vi "CANOpen_Main.vi"() -> ()   [LabVIEW 2021, in "CANOpen Addon Engine.lvlib"]
uses:
  CANOpen Addon Engine.lvlib
  SubVIS/CANOpen_Settings.ctl
  SubVIS/CANOpen_Node Settings.ctl
  Shared/CANOpen_Bus Settings.ctl
  Shared/CANOpen Interface Name.ctl
  <vilib>/CANopenLib/CANOPEN.llb/CANopen BaudRate.ctl
  SubVIS/CANOpen_Node Message Settings.ctl
  Shared/CANOpen_PDO Settings.ctl
  Shared/CANOpen_PDO Parameter Settings.ctl
  Shared/CANOpen_PDO Data Type.ctl
  Shared/CANopen Byte Order.ctl
  Shared/CANOpen_SDO Settings.ctl
  SubVIS/CANOpen_NMT Settings.ctl
  Shared/CanOpen_NMT_Config.ctl
  Shared/CanOpen_NMT_Static detect.ctl
  SubVIs/CanOpen_Main Node Ids.ctl
  SubVIS/CANOpen_VS Data Refs.ctl
  <vilib>/NI VeriStand/Custom Device API/Data Reference.ctl
  <vilib>/NI VeriStand/Custom Device API/Block Data Reference.ctl
  SubVIS/CANOpen_VS Bidirectional Data Refs.ctl
  SubVIS/CANOpen_VS SDOs Data Refs.ctl
  SubVIs/CanOpen_SDO Dynamic queue.ctl
  Shared/CANOpen_SDO queue W data.ctl
  Shared/CANOpen_SDO queue mode.ctl
  Shared/CANOpen_PDO Data Type in queue.ctl
  SubVIS/CANOpen_VS Status Management Data Refs.ctl
  SubVIs/CanOpen_NMT_HWOut_ChannelPairs.ctl
  SubVIs/CanOpen_NMT_HWIn_ChannelPairs.ctl
  <vilib>/NI VeriStand/Custom Device API/Custom Device Timed Loop Priority.ctl
  <vilib>/Platform/TimedLoop/XDataNode/timing_clust.ctl
  <vilib>/Platform/TimedLoop/XDataNode/nitl_modes.ctl
  <vilib>/Platform/TimedLoop/XDataNode/wakeup.ctl
  SubVIs/CanOpen_Main States.ctl
  SubVIs/CANOpen_Main_Close xPDOs.vi
  SubVIs/CANOpen_Main_Close HB NG EM.vi
  SubVIs/CANOpen_State_Opp_Preopp.vi
  SubVIs/CANOpen_Main_Compare RPDO Data for Change.vi
  <vilib>/CANopenLib/CANOPEN.llb/CANopen Interface Create.vi
  SubVIs/CANOpen_Check_Node_State for Node without HB NG.vi
  <vilib>/CANopenLib/CANOPEN.llb/CANopen Error Control Read.vi
  <vilib>/CANopenLib/CANOPEN.llb/CANopen Heartbeat State Read.vi
  <vilib>/CANopenLib/CANOPEN.llb/CANopen Node Guarding State Read.vi
  <vilib>/CANopenLib/CANOPEN.llb/CANopen Emergency Read.vi
  SubVIs/CANOpen_Main_Prepare status data.vi
  SubVIs/CANOpen_Main_Scale RPDO Data.vi
  <vilib>/CANopenLib/CANOPEN.llb/CANopen RPDO Write.vi
  <vilib>/CANopenLib/CANOPEN.llb/CANopen TPDO Read.vi
  SubVIs/CANOpen_Main_Scale TPDO Data.vi
  <vilib>/CANopenLib/CANOPEN.llb/CANopen Close.vi
  <vilib>/CANopenLib/CANOPEN.llb/CANopen SYNC Close.vi
  <vilib>/CANopenLib/CANOPEN.llb/CANopen RPDO Close.vi
  <vilib>/CANopenLib/CANOPEN.llb/CANopen TPDO Close.vi
  <vilib>/CANopenLib/CANOPEN.llb/CANopen SDO Create.vi
  <vilib>/CANopenLib/CANOPEN.llb/CANopen SDO Write.vi
  <vilib>/CANopenLib/CANOPEN.llb/CANopen SDO Write [U16].vi
  <vilib>/CANopenLib/CANOPEN.llb/CANopen SDO Close.vi
  <vilib>/CANopenLib/CANOPEN.llb/CANopen Heartbeat Close.vi
  <vilib>/CANopenLib/CANOPEN.llb/CANopen SDO Write [U8].vi
  <vilib>/CANopenLib/CANOPEN.llb/CANopen Node Guarding Close.vi
  <vilib>/CANopenLib/CANOPEN.llb/CANopen Emergency Close.vi
  SubVIs/CANOpen_Main_Set All Node States.vi
  <vilib>/CANopenLib/CANOPEN.llb/CANopen Interface Close.vi
  <vilib>/Platform/TimedLoop/XDataNode/XDataNode.xnode
  <vilib>/Platform/TimedLoop/XDataNode/XDNodeRunTimeDep.lvlib
  <vilib>/NI VeriStand/Custom Device API/Custom Device API.lvlib
  Shared/CANOpen Addon Shared.lvlib
panel:
  out "Interface Name":T1 caption="CANOpen Interface Name" items=["CANopen01", "CANopen02", "CANopen03", "CANopen04", "CANopen05", "CANopen06", "CANopen07", "CANopen08", "CANopen09", "CANopen10", "CANopen11", "CANopen12", "CANopen13", "CANopen14", "CANopen15", "CANopen16", "CANopen17", "CANopen18", "CANopen19", "CANopen20", "CANopen21", "CANopen22", "CANopen23", "CANopen24", "CANopen25", "CANopen26", "CANopen27", "CANopen28", "CANopen29", "CANopen30", "CANopen31", "CANopen32"]
  in  "Parent":string
  in  "Parameters":T2={"Driver Settings"={"CANOpen Bus Settings"={"CANOpen Interface Name"=0, "Baud Rate"=0, "Termination"=FALSE, "Sync Period (ms)"=10, "Enable 9881"=FALSE, "RIO Device"=0, "Enable SYNC"=FALSE, "Scan & Print"=FALSE}, "Nodes"=[], "Node Ids"=[]}, "Data References"={"Hardware Input"={"FIFO"=refnum, "Channel Pairs"={"Chan Refs"=[], "Prev. Values"=[]}}, "Hardware Output"={"FIFO"=refnum, "Channel Pairs"={"Block Refs"=[], "Prev. Values"=[]}}}, "Bus Commands"={"Hardware Output"={"FIFO"=refnum, "Channel Pairs"={"Chan Refs"=[], "Prev. Values"=[]}}, "Hardware Input"={"FIFO"=refnum}}, "SDO Asynch"={"List SDO"={"FIFO Req"=refnum, "Req Chan."={"Chan Refs"=[], "NodeIndex"=[]}, "FIFO Resp"=refnum, "Resp Chan."={"Chan Refs"=[]}, "Node IDs"=[], "FIFO array"=[]}, "HW Dyn Write"={"FIFO Req"=refnum, "FIFO Resp"=refnum, "Req Chan."={"Chan Refs"=[], "Node IDs"=[]}, "Resp Chan."={"Chan Refs"=[]}}, "HW Dyn Read"={"FIFO Req"=refnum, "FIFO Resp"=refnum, "Req Chan."={"Chan Refs"=[], "Node IDs"=[]}, "Resp Chan."={"Chan Refs"=[]}}}, "Status NMT"={"Hardware Output"={"FIFO"=refnum, "Channel Pairs"={"Chan Refs"=[], "Prev. Values"=[], "Node index"=[]}}, "Hardware Input"={"FIFO"=refnum, "Channel Pairs"={"Chan Refs"=[], "Prev. Values"=[], "Node index"=[]}}}} {"Status NMT"."Hardware Output"."Channel Pairs"."Chan Refs"."Data Reference" format="%.0x"; "Status NMT"."Hardware Input"."Channel Pairs"."Chan Refs" format="%.0x"; "SDO Asynch"."HW Dyn Read"."Resp Chan."."Chan Refs" format="%.0x"; "SDO Asynch"."HW Dyn Read"."Req Chan."."Chan Refs" format="%.0x"; "SDO Asynch"."HW Dyn Write"."Resp Chan."."Chan Refs" format="%.0x"; "SDO Asynch"."HW Dyn Write"."Req Chan."."Chan Refs" format="%.0x"; "SDO Asynch"."List SDO"."Resp Chan."."Chan Refs" format="%.0x"; "SDO Asynch"."List SDO"."Req Chan."."Chan Refs" format="%.0x"; "Bus Commands"."Hardware Output"."Channel Pairs"."Chan Refs" format="%.0x"; "Data References"."Hardware Input"."Channel Pairs"."Chan Refs" format="%.0x"; "Data References"."Hardware Output"."Channel Pairs"."Block Refs"."Data Reference" format="%.0x"; "Driver Settings"."CANOpen Bus Settings"."Baud Rate" items=["1 Mbit/s"=0, "800 kbit/s"=1, "500 kbit/s"=2, "250 kbit/s"=3, "125 kbit/s"=4, "50 kbit/s"=6, "20 kbit/s"=7, "10 kbit/s"=8]; "Driver Settings"."CANOpen Bus Settings"."CANOpen Interface Name" items=["CANopen01", "CANopen02", "CANopen03", "CANopen04", "CANopen05", "CANopen06", "CANopen07", "CANopen08", "CANopen09", "CANopen10", "CANopen11", "CANopen12", "CANopen13", "CANopen14", "CANopen15", "CANopen16", "CANopen17", "CANopen18", "CANopen19", "CANopen20", "CANopen21", "CANopen22", "CANopen23", "CANopen24", "CANopen25", "CANopen26", "CANopen27", "CANopen28", "CANopen29", "CANopen30", "CANopen31", "CANopen32"]; "Driver Settings"."Nodes"."NMT"."Node init static SDO state" items=["start remote node"=1, "enter pre-operational"=128]; "Driver Settings"."Nodes"."NMT"."Node run state" items=["start remote node"=1, "stop remote node"=2, "enter pre-operational"=128, "reset node"=129, "reset communication"=130]; "Driver Settings"."Nodes"."Dynamic SDOs"."Sub-Index (0)" format="%.0x"; "Driver Settings"."Nodes"."Dynamic SDOs"."Object Index" format="%.0x"; "Driver Settings"."Nodes"."Dynamic SDOs"."Block Data" format="%.0x"; "Driver Settings"."Nodes"."RPDOs"."PDO Channel" items=["PDO 1", "PDO 2", "PDO 3", "PDO 4"]; "Driver Settings"."Nodes"."TPDOs"."PDO Channel" items=["PDO 1", "PDO 2", "PDO 3", "PDO 4"]; "Driver Settings"."Nodes"."SDOs"."Sub-Index (0)" format="%.0x"; "Driver Settings"."Nodes"."SDOs"."Object Index" format="%.0x"; "Driver Settings"."Nodes"."SDOs"."Block Data" format="%.0x"}
  in  "stop":bool
  in  "error in":errorcluster
  out "error out":errorcluster
  # "LSB"
  # "MSB"
  # "LSB"
  # "MSB"
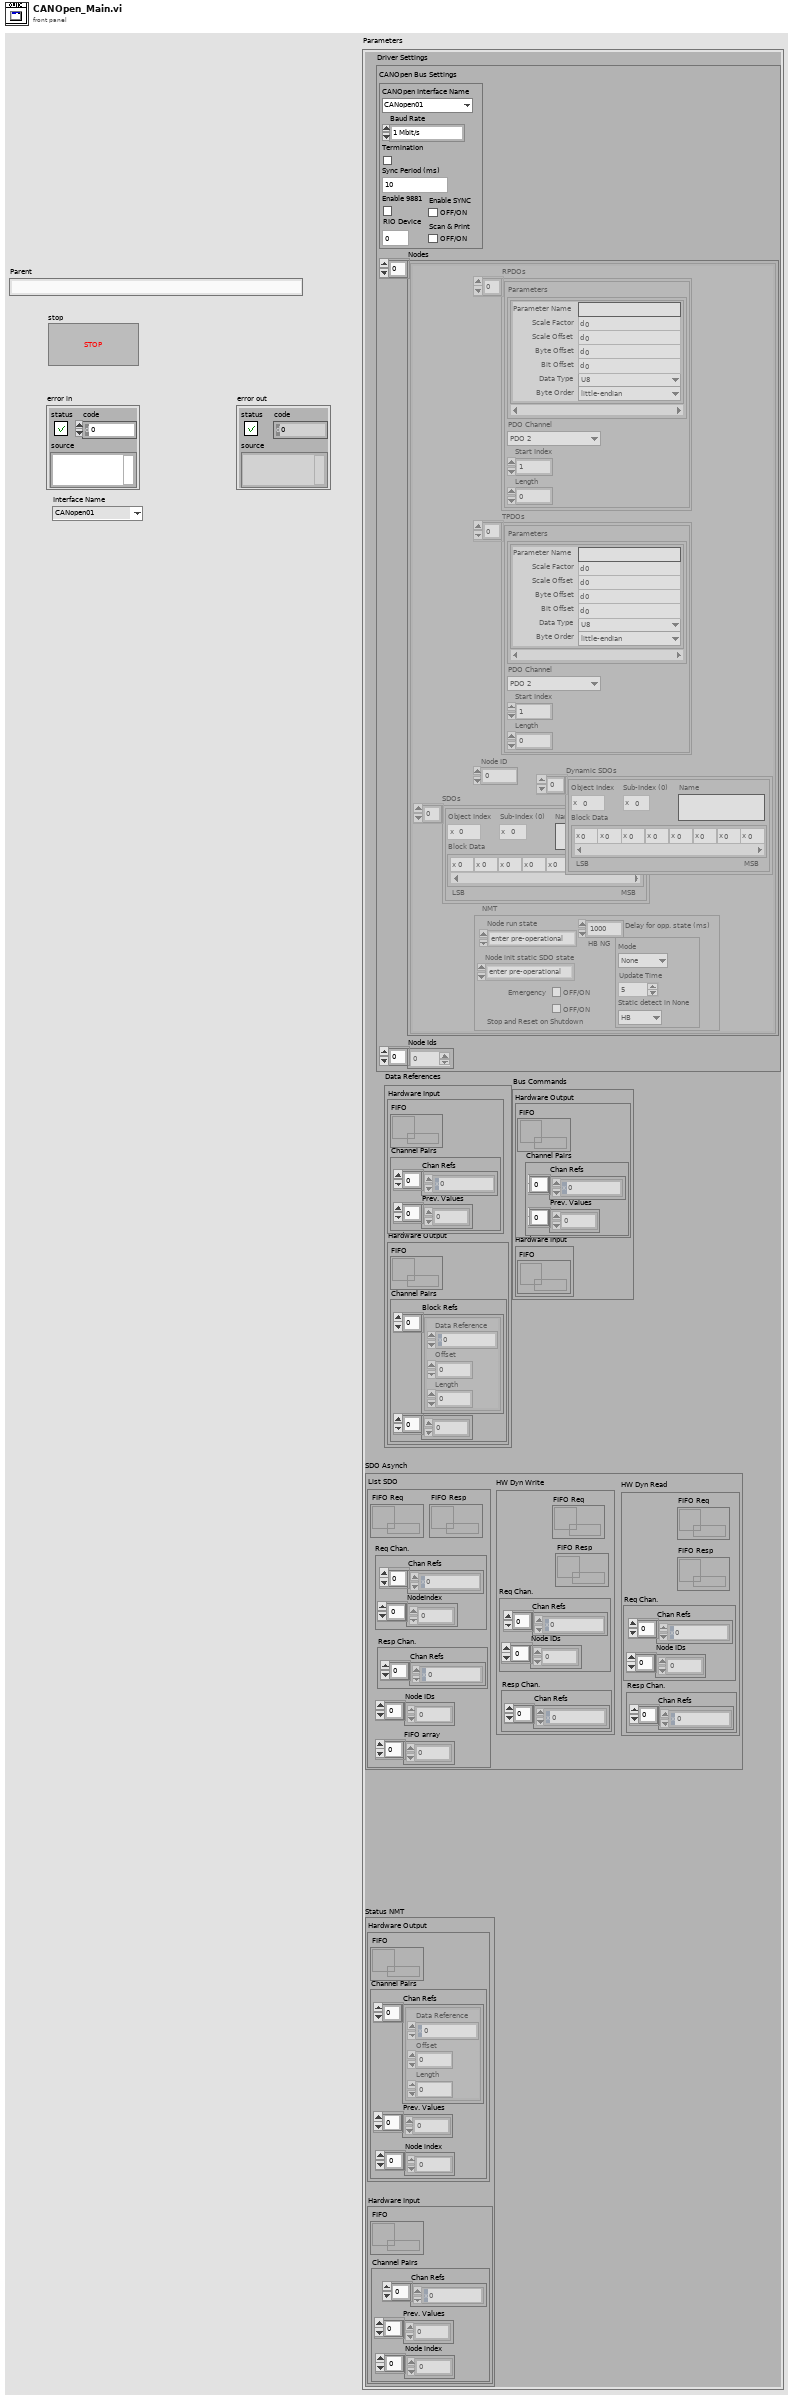
[diagram p1: front panel]
types:
  T1 = typedef "CANOpen Addon Shared.lvlib/CANOpen Interface Name.ctl" = u32
  T2 = typedef "CANOpen Addon Engine.lvlib/CANOpen_Settings.ctl" = cluster{"Driver Settings":T3, "Data References":T16, "Bus Commands":T19, "SDO Asynch":T20, "Status NMT":T21}
  T3 = typedef "CANOpen Addon Engine.lvlib/CANOpen_Node Settings.ctl" = cluster{"CANOpen Bus Settings":T4, "Nodes":T6[], "Node Ids":T15}
  T4 = typedef "CANOpen Addon Shared.lvlib/CANOpen_Bus Settings.ctl" = cluster{"CANOpen Interface Name":T1, "Baud Rate":T5, "Termination":bool, "Sync Period (ms)":i64, "Enable 9881":bool, "RIO Device":u16, "Enable SYNC":bool, "Scan & Print":bool}
  T5 = typedef "CANopen BaudRate.ctl" = u32
  T6 = typedef "CANOpen Addon Engine.lvlib/CANOpen_Node Message Settings.ctl" = cluster{"RPDOs":T7[], "TPDOs":T7[], "Node ID":u8, "SDOs":T11[], "Dynamic SDOs":T11[], "NMT":T12}
  T7 = typedef "CANOpen Addon Shared.lvlib/CANOpen_PDO Settings.ctl" = cluster{"Parameters":T8[], "PDO Channel":u8, "Start Index":u32, "Length":u32}
  T8 = typedef "CANOpen Addon Shared.lvlib/CANOpen_PDO Parameter Settings.ctl" = cluster{"Parameter Name":string, "Scale Factor":dbl, "Scale Offset":dbl, "Byte Offset":u8, "Bit Offset":u8, "Data Type":T9, "Byte Order":T10}
  T9 = typedef "CANOpen Addon Shared.lvlib/CANOpen_PDO Data Type.ctl" = enum16{"U8", "U16", "U32", "I8", "I16", "I32", "Single", "Double", "Boolean"}
  T10 = typedef "CANOpen Addon Shared.lvlib/CANopen Byte Order.ctl" = enum16{"big-endian network order", "little-endian"}
  T11 = typedef "CANOpen Addon Shared.lvlib/CANOpen_SDO Settings.ctl" = cluster{"Object Index":u16, "Sub-Index (0)":u8, "Block Data":u8[], "Name":string}
  T12 = typedef "CANOpen Addon Engine.lvlib/CANOpen_NMT Settings.ctl" = cluster{"Node run state":u16, "Emergency":bool, "HB NG":T13, "Delay for opp. state (ms)":dbl, "Node init static SDO state":u16, "Stop and Reset on Shutdown":bool}
  T13 = typedef "CANOpen Addon Shared.lvlib/CanOpen_NMT_Config.ctl" = cluster{"Mode":T14, "Update Time":u16, "Static detect in None":T14}
  T14 = typedef "CANOpen Addon Shared.lvlib/CanOpen_NMT_Static detect.ctl" = enum16{"None", "HB", "NG"}
  T15 = typedef "CANOpen Addon Engine.lvlib/CanOpen_Main Node Ids.ctl" = u8[]
  T16 = typedef "CANOpen Addon Engine.lvlib/CANOpen_VS Data Refs.ctl" = cluster{"Hardware Input":cluster{"FIFO":refnum<k33>, "Channel Pairs":cluster{"Chan Refs":T17[], "Prev. Values":dbl[]}}, "Hardware Output":cluster{"FIFO":refnum<k33>, "Channel Pairs":cluster{"Block Refs":T18[], "Prev. Values":dbl[]}}}
  T17 = typedef "Custom Device API.lvlib/Data Reference.ctl" = i32
  T18 = typedef "Custom Device API.lvlib/Block Data Reference.ctl" = cluster{"Data Reference":T17, "Offset":u64, "Length":u64}
  T19 = typedef "CANOpen Addon Engine.lvlib/CANOpen_VS Bidirectional Data Refs.ctl" = cluster{"Hardware Output":cluster{"FIFO":refnum<k33>, "Channel Pairs":cluster{"Chan Refs":T17[], "Prev. Values":dbl[]}}, "Hardware Input":cluster{"FIFO":refnum<k33>}}
  T20 = typedef "CANOpen Addon Engine.lvlib/CANOpen_VS SDOs Data Refs.ctl" = cluster{"List SDO":cluster{"FIFO Req":refnum<k33>, "Req Chan.":cluster{"Chan Refs":T17[], "NodeIndex":dbl[]}, "FIFO Resp":refnum<k33>, "Resp Chan.":cluster{"Chan Refs":T17[]}, "Node IDs":u8[], "FIFO array":dbl[]}, "HW Dyn Write":cluster{"FIFO Req":refnum<k33>, "FIFO Resp":refnum<k33>, "Req Chan.":cluster{"Chan Refs":T17[], "Node IDs":u8[]}, "Resp Chan.":cluster{"Chan Refs":T17[]}}, "HW Dyn Read":cluster{"FIFO Req":refnum<k33>, "FIFO Resp":refnum<k33>, "Req Chan.":cluster{"Chan Refs":T17[], "Node IDs":u8[]}, "Resp Chan.":cluster{"Chan Refs":T17[]}}}
  T21 = typedef "CANOpen Addon Engine.lvlib/CANOpen_VS Status Management Data Refs.ctl" = cluster{"Hardware Output":cluster{"FIFO":refnum<k33>, "Channel Pairs":T22}, "Hardware Input":cluster{"FIFO":refnum<k33>, "Channel Pairs":T23}}
  T22 = typedef "CANOpen Addon Engine.lvlib/CanOpen_NMT_HWOut_ChannelPairs.ctl" = cluster{"Chan Refs":T18[], "Prev. Values":dbl[], "Node index":dbl[]}
  T23 = typedef "CANOpen Addon Engine.lvlib/CanOpen_NMT_HWIn_ChannelPairs.ctl" = cluster{"Chan Refs":T17[], "Prev. Values":dbl[], "Node index":dbl[]}
  T24 = typedef "Custom Device API.lvlib/Custom Device Timed Loop Priority.ctl" = enum32{"Low", "Medium", "High"}
  T25 = typedef "CANOpen Addon Engine.lvlib/CanOpen_SDO queue ref.ctl" = cluster{"SDOReq":refnum<queue>}
  T26 = typedef "CANOpen Addon Engine.lvlib/CanOpen_Main States.ctl" = enum16{"NMT", "Device Status", "RPDO", "DYN SDO", "SYNC", "TPDO", "Status"}
  T27 = typedef "XDNodeRunTimeDep.lvlib/timing_clust.ctl" = cluster{"Expected End [f-1]":u64, "Actual End [f-1]":u64, "Finished Late? [f-1]":bool, "Expected End [i-1]":u64, "Actual End [i-1]":u64, "Finished Late? [i-1]":bool, "Expected Start [i]":u64, "Actual Start [i]":u64, "Expected Start [f]":u64, "Actual Start [f]":u64, "Source Name":string, "Structure Name":string, "Period":i64, "Deadline":i64, "Offset":i64, "Start":i64, "Priority":i32, "Timeout":i32, "Mode":T28, "Wakeup Reason":T29, "Error":errorcluster, "Source Type":string, "Secondary Source Type":string, "Global End Time":u64, "Global Start Time":u64, "Frame Duration":u64, "Iteration Duration":u64, "Assigned CPU":i32, "I/O Scan Engine Mode":u32}
  T28 = typedef "XDNodeRunTimeDep.lvlib/nitl_modes.ctl" = enum32{"No Change", "Process missed periods, maintain original phase", "Discard missed periods, maintain original phase", "Process missed periods, ignore original phase", "Discard missed periods, ignore original phase"}
  T29 = typedef "XDNodeRunTimeDep.lvlib/wakeup.ctl" = enum32{"Normal", "Aborted", "Asynchronous wakeup", "Timing source error", "Timed loop error", "Timeout"}
  T30 = typedef "CANOpen Addon Engine.lvlib/CANOpen_xPDO Refs.ctl" = cluster{"RPDOs":T31[], "TPDOs":T32[]}
  T31 = typedef "CANOpen Addon Engine.lvlib/CanOpen_RPDO Refs.ctl" = cluster{"RPDO Refs":refnum<k20>[]}
  T32 = typedef "CANOpen Addon Engine.lvlib/CanOpen_TPDO Refs.ctl" = cluster{"TPDO Refs":refnum<k20>[]}
  T33 = typedef "CANOpen Addon Engine.lvlib/CANOpen_HB_NG_EM Refs.ctl" = cluster{"HB Refs":refnum<k20>[], "NG Refs":refnum<k20>[], "EM Refs":refnum<k20>[], "Node ID":u8[]}
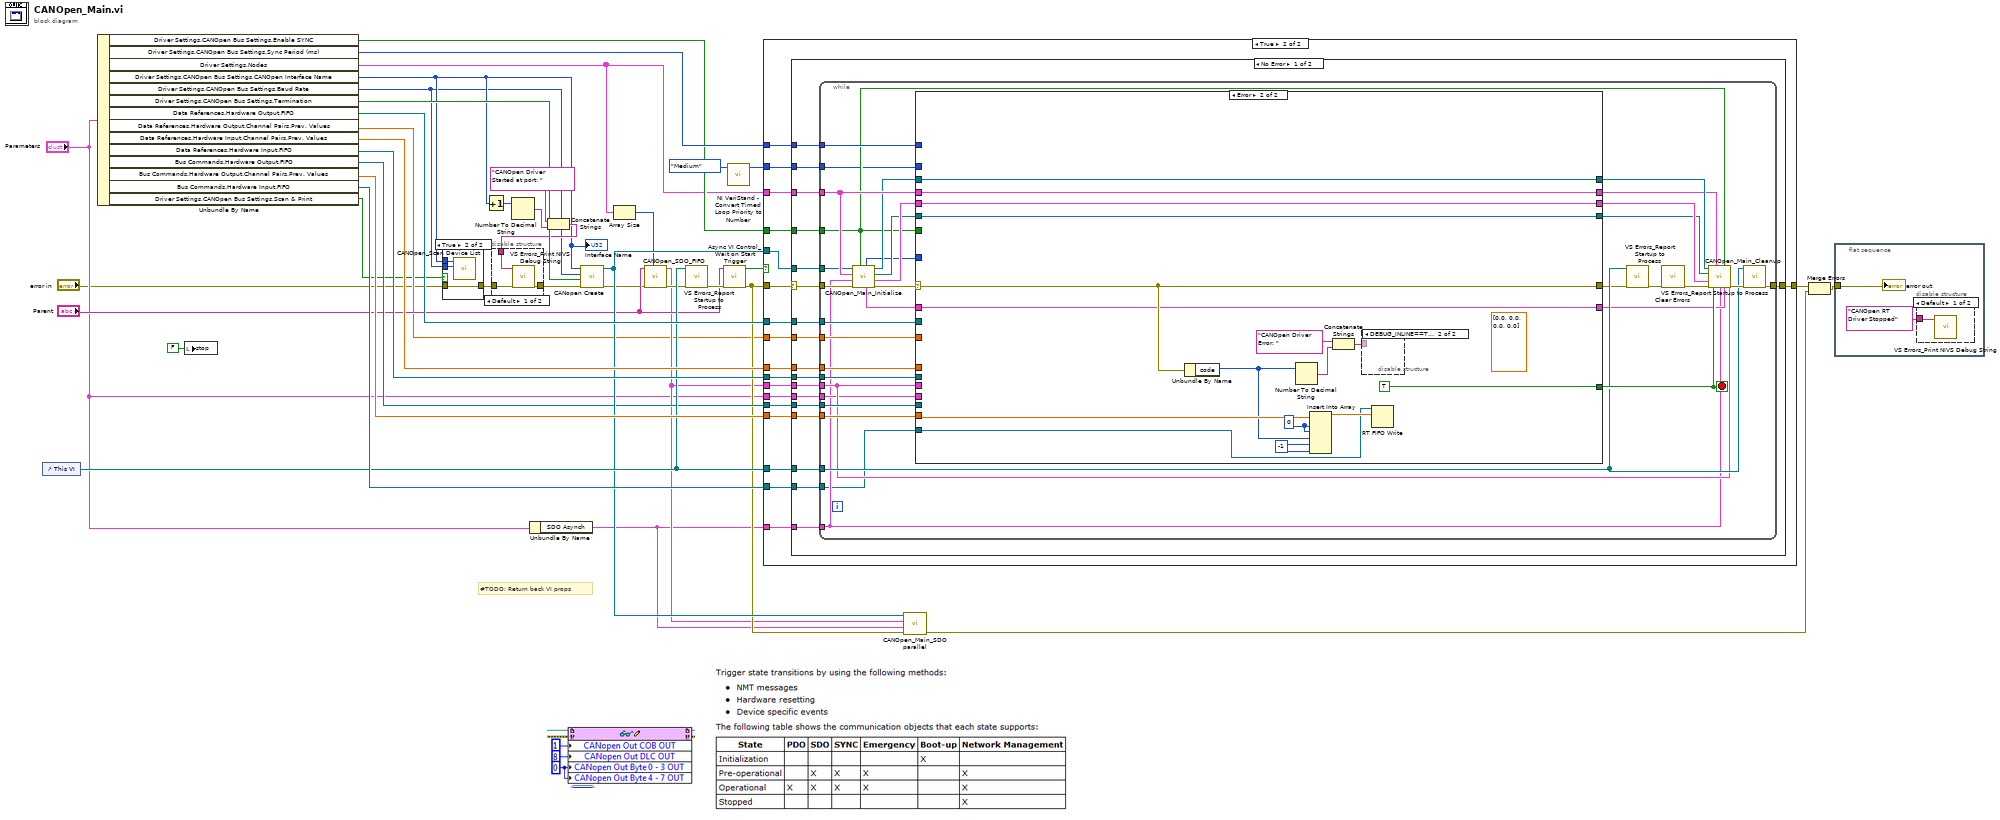
[diagram p0: block diagram]
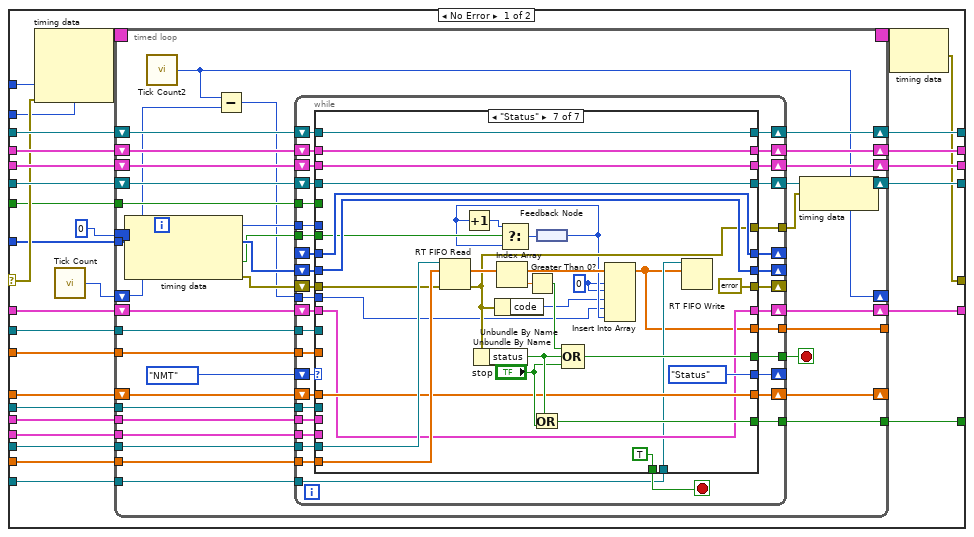
[diagram p5: hidden frame]
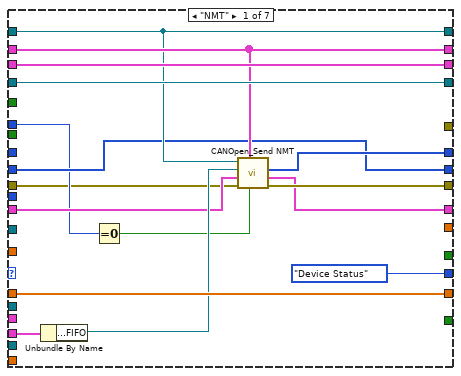
[diagram p6: hidden frame]
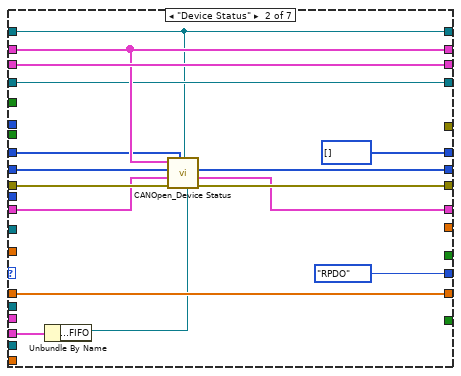
[diagram p7: hidden frame]
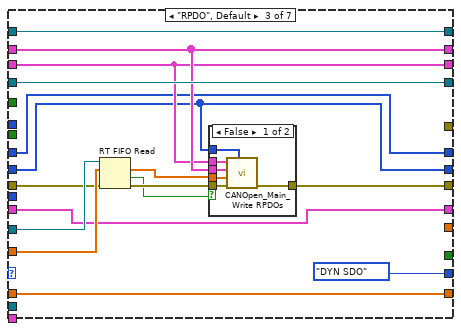
[diagram p8: hidden frame]
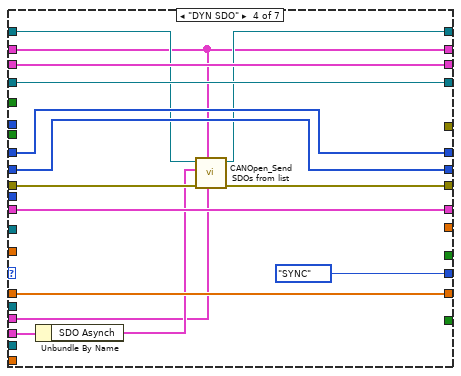
[diagram p10: hidden frame]
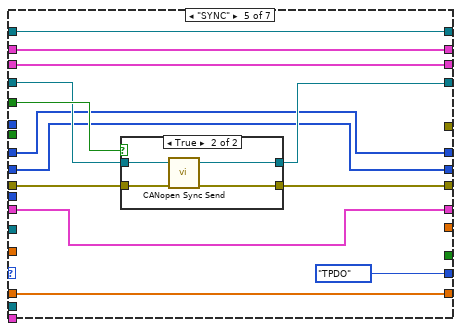
[diagram p11: hidden frame]
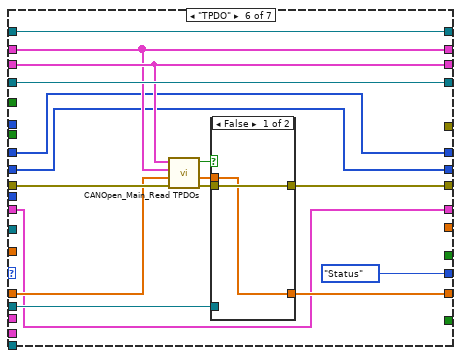
[diagram p13: hidden frame]
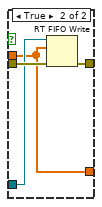
[diagram p14: hidden frame]
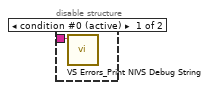
[diagram p15: hidden frame]
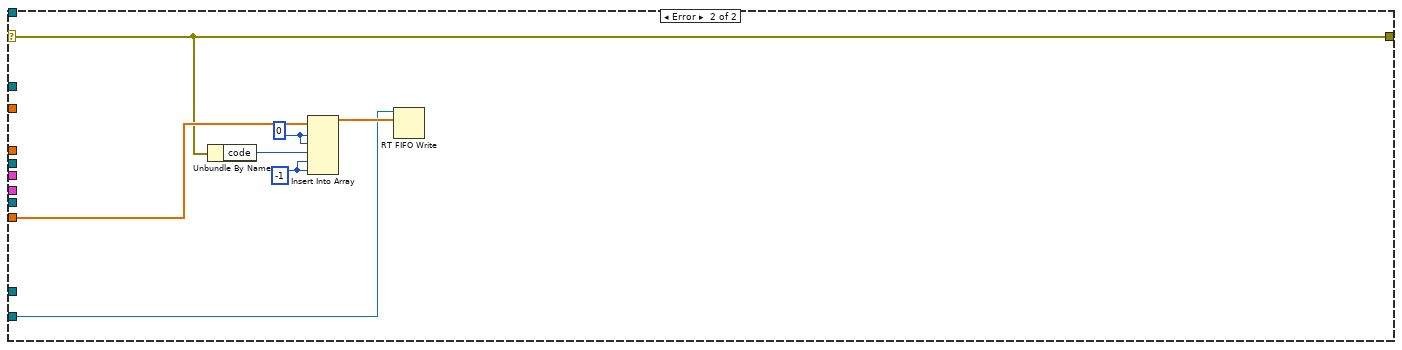
[diagram p16: hidden frame]
diagram:
  # "#TODO: Return back VI props"
  n1 = control-ref of="This VI"() -> (w28:refnum<vi>)
  n2 = Unbundle By Name("Parameters") -> ("Driver Settings.CANOpen Bus Settings.Enable SYNC"=w18:bool, "Driver Settings.CANOpen Bus Settings.Sync Period (ms)"=w35:i64, "Driver Settings.Nodes"=w10:T6[], "Driver Settings.CANOpen Bus Settings.CANOpen Interface Name"=w2:T1, "Driver Settings.CANOpen Bus Settings.Baud Rate"=w1:T5, "Driver Settings.CANOpen Bus Settings.Termination"=w39:bool, "Data References.Hardware Output.FIFO"=w36:refnum<k33>, "Data References.Hardware Output.Channel Pairs.Prev. Values"=w6:dbl[], "Data References.Hardware Input.Channel Pairs.Prev. Values"=w38:dbl[], "Data References.Hardware Input.FIFO"=w37:refnum<k33>, "Bus Commands.Hardware Output.FIFO"=w19:refnum<k33>, "Bus Commands.Hardware Output.Channel Pairs.Prev. Values"=w34:dbl[], "Bus Commands.Hardware Input.FIFO"=w33:refnum<k33>, "Driver Settings.CANOpen Bus Settings.Scan & Print"=w3:bool)
  "Interface Name" <- w2
  n3 = local write "stop"(FALSE ("stop")) -> ()
  n4 = case shown="True" w3 {
    tunnel: [w40 w43] -> w5
    tunnel: "error in" -> [w40 w43]
    tunnel: w2 -> [_ w42]
    tunnel: w1 -> [_ w41]
    frame False {
    }
    frame True {
      n5 = call "CANOpen_Scan Device List.vi"("Baud Rate"=w41, "CANOpen Interface Name"=w42) -> ()  [unwired: 10 in]
    }
  }
  n6 = Increment(x=w2) -> (x+1=w27:T1)
  n7 = Number To Decimal String(number=w27) -> (decimal integer string=w26:string)  [unwired: 1 in]
  n8 = Unbundle By Name("Parameters") -> ("SDO Asynch"=w7:T20)
  n9 = Concatenate Strings("CANOpen Driver Started at port: " ("Debug String"), w26) -> (w24:string)
  n10 = disable-structure shown="Default" {
    disable-tunnel: [w46 w47] -> w32
    disable-tunnel: w24 -> [w45 _]
    disable-tunnel: w5 -> [w44 w47]
    frame condition #0 (active) {
      n11 = call "VS Errors_Print NIVS Debug String.vi"("error in (no error)"=w44, "Debug String"=w45) -> ("error out"=w46:errorcluster)  [unwired: 8 in]
    }
    frame condition #1 {
    }
  }
  n12 = call-poly <vilib>:"CANopen Create.vi"("error in (no error)"=w32, "termination? (F)"=w39, "baud rate"=w1, "interface name"=w2) -> ("error out"=w14:errorcluster, "interface object out"=w21:refnum<k20>)  [unwired: 6 in]
  n13 = Array Size(array=w10) -> (size(s)=w9:i32)
  n14 = call "CANOpen_SDO_FIFO.vi"("nodes"=w9, "error in"=w14, "Parent"="Parent") -> ("error out"=w15:errorcluster, "SDO queues"=w11:T25)  [unwired: 7 in]
  n15 = call "VS Errors_Report Startup to Process.vi"("Error"=w15, "This VI"=w28) -> ("error out"=w29:errorcluster)  [unwired: 9 in]
  n16 = call "Async VI Control_Wait on Start Trigger.vi"("error in (no error)"=w29, "Name"="Parent") -> ("error out"=w16:errorcluster, "notification"=w30:bool)  [unwired: 8 in]
  n17 = call <vilib>:"NI VeriStand - Convert Timed Loop Priority to Number.vi"("Priority"=Custom_Device_Timed_Loop_Priority."Medium") -> ("Numeric Priority"=w12:i32)  [unwired: 10 in]
  n18 = case shown="True" w30 {
    tunnel: w21 -> [_ w66]
    tunnel: w10 -> [_ w65]
    tunnel: w38 -> [_ w64]
    tunnel: w37 -> [_ w63]
    tunnel: w36 -> [_ w62]
    tunnel: w6 -> [_ w61]
    tunnel: w35 -> [_ w60]
    tunnel: w19 -> [_ w59]
    tunnel: w34 -> [_ w58]
    tunnel: w33 -> [_ w57]
    tunnel: [w48 w56] -> w31
    tunnel: w28 -> [_ w55]
    tunnel: w16 -> [w48 w54]
    tunnel: w18 -> [_ w53]
    tunnel: w11 -> [_ w52]
    tunnel: "Parameters" -> [_ w51]
    tunnel: w12 -> [_ w50]
    tunnel: w7 -> [_ w49]
    frame False {
    }
    frame True {
      n19 = case shown="No Error" w54 {
        selector: w54 -> [w73 w393]
        tunnel: w66 -> [w84 _]
        tunnel: w65 -> [w83 _]
        tunnel: w64 -> [w82 _]
        tunnel: w63 -> [w81 _]
        tunnel: w62 -> [w80 _]
        tunnel: w61 -> [w79 _]
        tunnel: w60 -> [w78 _]
        tunnel: w59 -> [w77 _]
        tunnel: w58 -> [w76 w395]
        tunnel: w57 -> [w75 w394]
        tunnel: [w72 w393] -> w56
        tunnel: w55 -> [w74 _]
        tunnel: w53 -> [w71 _]
        tunnel: w52 -> [w70 _]
        tunnel: w51 -> [w69 _]
        tunnel: w50 -> [w68 _]
        tunnel: w49 -> [w67 _]
        frame No Error {
          n20 = while {
            tunnel: w73 -> [w104]
            tunnel: w84 -> [w105]
            tunnel: [w98] -> w72
            tunnel: w83 -> [w106]
            tunnel: w82 -> [w117]
            tunnel: w81 -> [w118]
            tunnel: w75 -> [w86]
            tunnel: w80 -> [w116]
            tunnel: w79 -> [w115]
            tunnel: w77 -> [w114]
            tunnel: w76 -> [w113]
            tunnel: w78 -> [w112]
            tunnel: w74 -> [w97]
            tunnel: w71 -> [w96]
            tunnel: w70 -> [w92]
            tunnel: w69 -> [w91]
            tunnel: w68 -> [w90]
            tunnel: w67 -> [w89]
            stop <- w107 stop-if-true
            n21 = call "CANOpen_Main_Initialize.vi"("Enable SYNC"=w96, "error in (no error)"=w104, "SDO Asynch"=w89, "Nodes"=w106, "interface object"=w105) -> ("error out"=w100:errorcluster, "xPDO Refs"=w103:T30, "SYNC object out"=w101:refnum<k20>, "interface object out"=w102:refnum<k20>, "Security Ref"=w94:T33, "Node States"=w95:u16[])  [unwired: 1 in]
            n22 = case shown="Error" w100 {
              selector: w100 -> [w129 w384]
              tunnel: w118 -> [w146 _]
              tunnel: w117 -> [w145 _]
              tunnel: w116 -> [w144 _]
              tunnel: w115 -> [w143 _]
              tunnel: w114 -> [w142 _]
              tunnel: w113 -> [w141 w379]
              tunnel: w112 -> [w140 _]
              tunnel: [w139 w387] -> w111
              tunnel: [w138 w388] -> w110
              tunnel: [w137 w385] -> w109
              tunnel: [w136 w386] -> w108
              tunnel: [w135 TRUE] -> w107
              tunnel: w106 -> [w134 w386]
              tunnel: w103 -> [w133 w387]
              tunnel: w102 -> [w132 w385]
              tunnel: w101 -> [w131 w388]
              tunnel: [w130 w384] -> w87
              tunnel: w96 -> [w128 _]
              tunnel: w95 -> [w127 _]
              tunnel: w94 -> [w126 w380]
              tunnel: [w125 w380] -> w93
              tunnel: w92 -> [w124 _]
              tunnel: w91 -> [w123 _]
              tunnel: w90 -> [w122 _]
              tunnel: w86 -> [w121 w374]
              frame No Error {
                n23 = node-c288(w140, w129, w122) -> (w148:T27)
                n24 = call "Tick Count"() -> ("Tick Count(mSec)"=w119:u32)
                n25 = timed-loop {
                  timing: w148 -> [_]
                  timing-out: [_] -> w147
                  shift-right: [w171] -> w138
                  shift-left: w131 -> [w174]
                  shift-right: [w170] -> w137
                  shift-left: w132 -> [w175]
                  tunnel: [w172] -> w135
                  shift-right: [w163] -> w139
                  shift-left: w133 -> [w165]
                  shift-right: [w164] -> w136
                  shift-left: w134 -> [w166]
                  tunnel: w146 -> [w167]
                  tunnel: w144 -> [w179]
                  tunnel: w143 -> [w178]
                  tunnel: w142 -> [w177]
                  tunnel: w141 -> [w176]
                  shift-right: [w168] -> _
                  shift-left: w145 -> [w180]
                  tunnel: w128 -> [w169]
                  tunnel: w127 -> [w158]
                  tunnel: w124 -> [w160]
                  tunnel: w123 -> [w159]
                  shift-right: [w161] -> w125
                  shift-left: w126 -> [w162]
                  tunnel: [w156] -> _
                  tunnel: w121 -> [w155]
                  border: u32 0 -> [_]
                  shift-right: [w151] -> _
                  shift-left: w119 -> [w150]
                  i -> [w157]
                  stop <- w181 stop-if-true
                  n26 = node-c288() -> (w153:bool, w154:errorcluster)  [unwired: 1 in, 1 out]
                  n27 = call "Tick Count2"() -> ("Tick Count(mSec)"=w151:u32)
                  n28 = Subtract(x=w151, y=w150) -> (x-y=w149:u32)
                  n29 = while {
                    tunnel: [w218] -> w181
                    tunnel: w179 -> [w215]
                    tunnel: w178 -> [w214]
                    tunnel: w177 -> [w213]
                    tunnel: w176 -> [w212]
                    shift-right: [w200] -> _
                    shift-left: CanOpen_Main_States."NMT" -> [w209]
                    tunnel: [w208] -> w172
                    shift-right: [w206] -> _
                    shift-left: w154 -> [w216]
                    shift-right: [w205] -> w171
                    shift-left: w174 -> [w210]
                    shift-right: [w204] -> w170
                    shift-left: w175 -> [w211]
                    tunnel: w169 -> [w203]
                    shift-right: [w202] -> w168
                    shift-left: w180 -> [w217]
                    tunnel: w167 -> [w201]
                    shift-right: [w197] -> w164
                    shift-left: w166 -> [w199]
                    shift-right: [w196] -> w163
                    shift-left: w165 -> [w198]
                    shift-right: [w193] -> _
                    shift-left: _ -> [w192]
                    tunnel: w160 -> [w191]
                    shift-right: [w190] -> _
                    shift-left: w158 -> [w189]
                    tunnel: w159 -> [w188]
                    shift-right: [w194] -> w161
                    shift-left: w162 -> [w195]
                    tunnel: w157 -> [w187]
                    tunnel: [w186] -> w156
                    tunnel: w155 -> [w185]
                    tunnel: w149 -> [w184]
                    tunnel: w153 -> [w183]
                    tunnel: [w182] -> w152
                    stop <- w207 stop-if-true
                    n30 = case shown="\"Status\"" w209 {
                      tunnel: [_ _ _ _ _ _ w360] -> w218
                      tunnel: [w234 w241 w260 w288 w297 w322 w350] -> w205
                      tunnel: w217 -> [w233 w250 w259 w287 w295 w316 w348]
                      tunnel: w216 -> [w219 w246 w252 w278 w300 w318 w351]
                      tunnel: w215 -> [_ _ w265 _ _ _ _]
                      tunnel: w214 -> [_ _ w266 _ _ _ _]
                      tunnel: w213 -> [_ _ _ _ _ _ w359]
                      tunnel: w212 -> [_ _ _ _ _ _ w358]
                      tunnel: [_ _ _ _ _ _ w354] -> w208
                      tunnel: w211 -> [w227 w240 w261 w280 w301 w323 w349]
                      tunnel: [w227 w240 w261 w279 w301 w323 w349] -> w204
                      tunnel: w210 -> [w234 w241 w260 w288 w298 w322 w350]
                      tunnel: [_ _ _ _ _ _ TRUE] -> w207
                      tunnel: [w231 w245 w251 w274 w296 w308 errorcluster {"status"=FALSE, "code"=0, "source"=""} ("error out")] -> w206
                      tunnel: w203 -> [_ _ _ _ w299 _ _]
                      tunnel: [w233 w250 w259 w287 w295 w317 w348] -> w202
                      tunnel: w201 -> [_ _ _ _ _ w315 _]
                      tunnel: [CanOpen_Main_States."Device Status" CanOpen_Main_States."RPDO" CanOpen_Main_States."DYN SDO" CanOpen_Main_States."SYNC" CanOpen_Main_States."TPDO" CanOpen_Main_States."Status" CanOpen_Main_States."Status"] -> w200
                      tunnel: w199 -> [w229 w247 w257 w275 w293 w312 w346]
                      tunnel: w198 -> [w232 w249 w256 w285 w292 w313 w345]
                      tunnel: [w229 w247 w257 w275 w293 w312 w346] -> w197
                      tunnel: [w232 w249 w256 w285 w292 w313 w345] -> w196
                      tunnel: w195 -> [w223 w244 w255 w284 w291 w311 w342]
                      tunnel: [w222 w243 w255 w284 w291 w311 w342] -> w194
                      tunnel: [w228 u8[] [] ("Node IDs to Check") w253 w283 w290 w310 w344] -> w193
                      tunnel: w192 -> [_ w235 w253 w283 w290 w310 w344]
                      tunnel: w191 -> [_ _ _ w276 _ _ _]
                      tunnel: [w224 w239 w254 w282 w289 w309 w339] -> w190
                      tunnel: w189 -> [w224 w236 w254 w282 w289 w309 w339]
                      tunnel: w188 -> [w226 w238 _ w281 _ _ _]
                      tunnel: w187 -> [w220 _ _ _ _ _ _]
                      tunnel: [_ _ _ _ _ _ w340] -> w186
                      tunnel: w185 -> [_ _ _ _ _ _ w341]
                      tunnel: w184 -> [_ _ _ _ _ _ w332]
                      tunnel: w183 -> [_ _ _ _ _ _ w338]
                      tunnel: [_ _ _ _ _ _ w335] -> w182
                      frame "NMT" {
                        n31 = Unbundle By Name(w226) -> ("Status NMT.Hardware Output.FIFO"=w225:refnum<k33>)
                        n32 = Equal To 0?(x=w220) -> (x = 0?=w221:bool)
                        n33 = call "CANOpen_Send NMT.vi"("Init check"=w221, "Nodes"=w229, "error in"=w219, "Security Ref in"=w223, "FIFO"=w225, "interface object"=w227) -> ("error out"=w231:errorcluster, "Security Ref out"=w222:T33, "Node IDs to Check"=w228:i16[])  [unwired: 2 in, 1 out]
                      }
                      frame "Device Status" {
                        n34 = Unbundle By Name(w238) -> ("Status NMT.Hardware Input.FIFO"=w237:refnum<k33>)
                        n35 = call "CANOpen_Device Status .vi"("Status NMT.Hardware Input.FIFO"=w237, "Node IDs to Check"=w235, "interface object in"=w240, "error in (no error)"=w246, "Security Ref in"=w244, "Node States"=w236, "Nodes"=w247) -> ("error out"=w245:errorcluster, "Security Ref out"=w243:T33, "Node States out"=w239:u16[])  [unwired: 2 in]
                      }
                      frame "RPDO", Default {
                        n36 = RT FIFO Read(0:w265, 1:w266, 3:w252) -> (9:w262:dbl[], 10:w263:bool, 11:w264:errorcluster)  [unwired: 1 in, 2 out]
                        n37 = case shown="False" w263 {
                          tunnel: [w272 w273] -> w251
                          tunnel: w264 -> [w271 w273]
                          tunnel: w262 -> [w270 _]
                          tunnel: w257 -> [w269 _]
                          tunnel: w256 -> [w268 _]
                          tunnel: w254 -> [w267 _]
                          frame False {
                            n38 = call "CANOpen_Main_Write RPDOs.vi"("Node states"=w267, "error in (no error)"=w271, "Data"=w270, "Nodes"=w269, "xPDO Refs"=w268) -> ("error out"=w272:errorcluster)  [unwired: 6 in]
                          }
                          frame True {
                          }
                        }
                      }
                      frame "DYN SDO" {
                        n39 = Unbundle By Name(w281) -> ("SDO Asynch"=w277:T20)
                        n40 = call "CANOpen_Send SDOs from list.vi"("SDO queues"=w276, "Nodes"=w275, "error in"=w278, "SDO Asynch"=w277, "interface object"=w280) -> ("error out"=w274:errorcluster, "interface object out"=w279:refnum<k20>)  [unwired: 5 in]
                      }
                      frame "SYNC" {
                        n41 = case shown="True" w299 {
                          tunnel: w300 -> [w302 w307]
                          tunnel: w298 -> [w303 w306]
                          tunnel: [w303 w305] -> w297
                          tunnel: [w302 w304] -> w296
                          frame False {
                          }
                          frame True {
                            n42 = call <vilib>:"CANopen Sync Send.vi"("error in (no error)"=w307, "SYNC object in"=w306) -> ("error out"=w304:errorcluster, "SYNC object out"=w305:refnum<k20>)  [unwired: 8 in]
                          }
                        }
                      }
                      frame "TPDO" {
                        n43 = call "CANOpen_Main_Read TPDOs.vi"("error in (no error)"=w318, "Initial Data Array"=w316, "Nodes"=w312, "xPDO Refs"=w313) -> ("error out"=w320:errorcluster, "Data Array"=w319:dbl[], "New Data?"=w321:bool)  [unwired: 5 in]
                        n44 = case shown="False" w321 {
                          tunnel: w319 -> [w324 w326]
                          tunnel: w320 -> [w325 w329]
                          tunnel: w315 -> [_ w328]
                          tunnel: [w325 w327] -> w308
                          tunnel: [w324 w326] -> w317
                          frame False {
                          }
                          frame True {
                            n45 = RT FIFO Write(0:w328, 1:w326, 3:w329) -> (11:w327:errorcluster)  [unwired: 2 in, 3 out]
                          }
                        }
                      }
                      frame "Status" {
                        w330 = 0 ("index")
                        n46 = RT FIFO Read(0:w359, 1:w358, 3:w351) -> (9:w343:dbl[], 11:w335:errorcluster)  [unwired: 1 in, 3 out]
                        n47 = Unbundle By Name(w335) -> ("status"=w356:bool)
                        n48 = Unbundle By Name(w335) -> ("code"=w331:i32)
                        n49 = Index Array(array=w343) -> (element=w357:dbl)  [unwired: 1 in]
                        n50 = Greater Than 0?(x=w357) -> (x > 0?=w353:bool)
                        n51 = Or(x=w356, y="stop") -> (x .or. y?=w354:bool)
                        n52 = feedback #1() -> (w333:u32)
                        n53 = Increment(x=w333) -> (x+1=w336:u32)
                        n54 = Select(t=w336, s=w338, f=w333) -> (s? t:f=w337:u32)
                        n55 = feedback-in #1(w337) -> ()
                        n56 = Compound Arithmetic op=OR(w353, w356, "stop") -> (w360:bool)
                        n57 = Insert Into Array(array=w343, index=w330, new element #1=w330, new element #2=w331, new element #3=w332, new element #4=w333) -> (w340:dbl[])
                        n58 = RT FIFO Write(0:w341, 1:w340) -> ()  [unwired: 3 in, 4 out]
                      }
                    }
                  }
                  n59 = node-c288(w152) -> ()  [unwired: 1 out]
                }
                n60 = node-c288(w147) -> (w130:errorcluster)
              }
              frame Error {
                w375 = -1 ("index")
                w377 = 0 ("index")
                (unwired) dbl[] [0.0, 0.0, 0.0, 0.0]
                n61 = Unbundle By Name(w384) -> ("code"=w376:i32)
                n62 = Number To Decimal String(number=w376) -> (decimal integer string=w382:string)  [unwired: 1 in]
                n63 = Insert Into Array(array=w379, index=w377, new element #1=w377, new element #2=w376, new element #3=w375, new element #4=w375) -> (w378:dbl[])
                n64 = Concatenate Strings("CANOpen Driver Error: " ("Debug String"), w382) -> (w381:string)
                n65 = disable-structure shown="DEBUG_INLINE==TRUE" {
                  disable-tunnel: w381 -> [w390 _]
                  frame condition #0 (active) {
                    n66 = call "VS Errors_Print NIVS Debug String.vi"("Debug String"=w390) -> ()  [unwired: 9 in, 1 out]
                  }
                  frame condition #1 {
                  }
                }
                n67 = RT FIFO Write(0:w374, 1:w378) -> ()  [unwired: 3 in, 4 out]
              }
            }
            n68 = call "VS Errors_Report Startup to Process.vi"("Error"=w87, "This VI"=w97) -> ("error out"=w88:errorcluster)  [unwired: 9 in]
            n69 = call <vilib>:"Clear Errors.vi"("error in (no error)"=w88) -> ("error out"=w85:errorcluster)  [unwired: 5 in, 1 out]
            n70 = call "CANOpen_Main_Cleanup.vi"("interface object"=w109, "Nodes"=w108, "Enable SYNC"=w96, "SYNC object in"=w110, "xPDO Refs"=w111, "SDO queues"=w92, "error in (no error)"=w85, "Exit"=w107, "SDO Asynch"=w89, "Security Ref"=w93) -> ("error out"=w99:errorcluster)  [unwired: 5 in]
            n71 = call "VS Errors_Report Startup to Process.vi"("Error"=w99, "This VI"=w97) -> ("error out"=w98:errorcluster)  [unwired: 9 in]
          }
        }
        frame Error {
          w391 = -1 ("index")
          w396 = 0 ("index")
          n72 = Unbundle By Name(w393) -> ("code"=w392:i32)
          n73 = Insert Into Array(array=w395, index=w396, new element #1=w396, new element #2=w392, new element #3=w391, new element #4=w391) -> (w397:dbl[])
          n74 = RT FIFO Write(0:w394, 1:w397) -> ()  [unwired: 3 in, 4 out]
        }
      }
    }
  }
  n75 = call "CANOpen_Main_SDO parallel.vi"("error in (no error)"=w16, "SDO Asynch"=w7, "SDO queues"=w11, "interface object in"=w21) -> ("error out"=w22:errorcluster)  [unwired: 7 in]
  n76 = Merge Errors(w31, w22) -> (w23:errorcluster)
  n77 = flat-sequence {
    tunnel: w23 -> [w398]
    frame #0 {
      n78 = disable-structure shown="Default" {
        disable-tunnel: "CANOpen RT Driver Stopped" ("Debug String") -> [w400 _]
        frame condition #0 (active) {
          n79 = call "VS Errors_Print NIVS Debug String.vi"("Debug String"=w400) -> ()  [unwired: 9 in, 1 out]
        }
        frame condition #1 {
        }
      }
      "error out" <- w398
    }
  }
